vi "test-discretizations.vi"() -> ()   [LabVIEW 2019]
uses:
  <vilib>/Analysis/Matrix/Datatypes/RealMatrix.ctl
  <vilib>/Rock Robotics/WPI/ThirdParty/JAS_Junk/TrajLib/MatBuilder_Create.vi
  <vilib>/Rock Robotics/WPI/ThirdParty/JAS_Junk/TrajLib/MatrixHelper_CoerceSize.vi
  <vilib>/Rock Robotics/WPI/ThirdParty/JAS_Junk/TrajLib/Trajectory_Library.lvlib
  <vilib>/Analysis/Matrix/NI_Matrix.lvlib
panel:
  out "CoVar 2":T1
  out "Cost 1":T1
  # "assertEquals(1.0, mat.get(0, 0), 1e-3);\n    assertEquals(0.0, mat.get(0, 1), 1e-3);\n    assertEquals(0.0, mat.get(0, 2), 1e-3);\n    assertEquals(0.0, mat.get(1, 0), 1e-3);\n    assertEquals(1.0 / 4.0, mat.get(1, 1), 1e-3);\n    assertEquals(0.0, mat.get(1, 2), 1e-3);\n    assertEquals(0.0, mat.get(0, 2), 1e-3);\n    assertEquals(0.0, mat.get(1, 2), 1e-3);\n    assertEquals(1.0 / 9.0, mat.get(2, 2), 1e-3);"
  # "assertEquals(1.0, mat.get(0, 0), 1e-3);\n    assertEquals(0.0, mat.get(0, 1), 1e-3);\n    assertEquals(0.0, mat.get(0, 2), 1e-3)\n;\n    assertEquals(0.0, mat.get(1, 0), 1e-3);\n    assertEquals(4.0, mat.get(1, 1), 1e-3);\n    assertEquals(0.0, mat.get(1, 2), 1e-3);\n\n    assertEquals(0.0, mat.get(0, 2), 1e-3);\n    assertEquals(0.0, mat.get(1, 2), 1e-3);\n    assertEquals(9.0, mat.get(2, 2), 1e-3);"
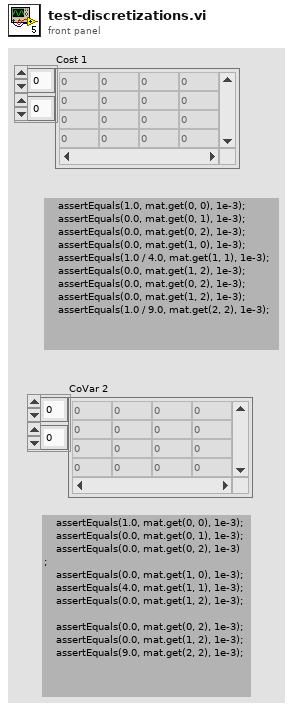
[diagram p1: front panel]
types:
  T1 = typedef "NI_Matrix.lvlib/RealMatrix.ctl" = dbl[][]
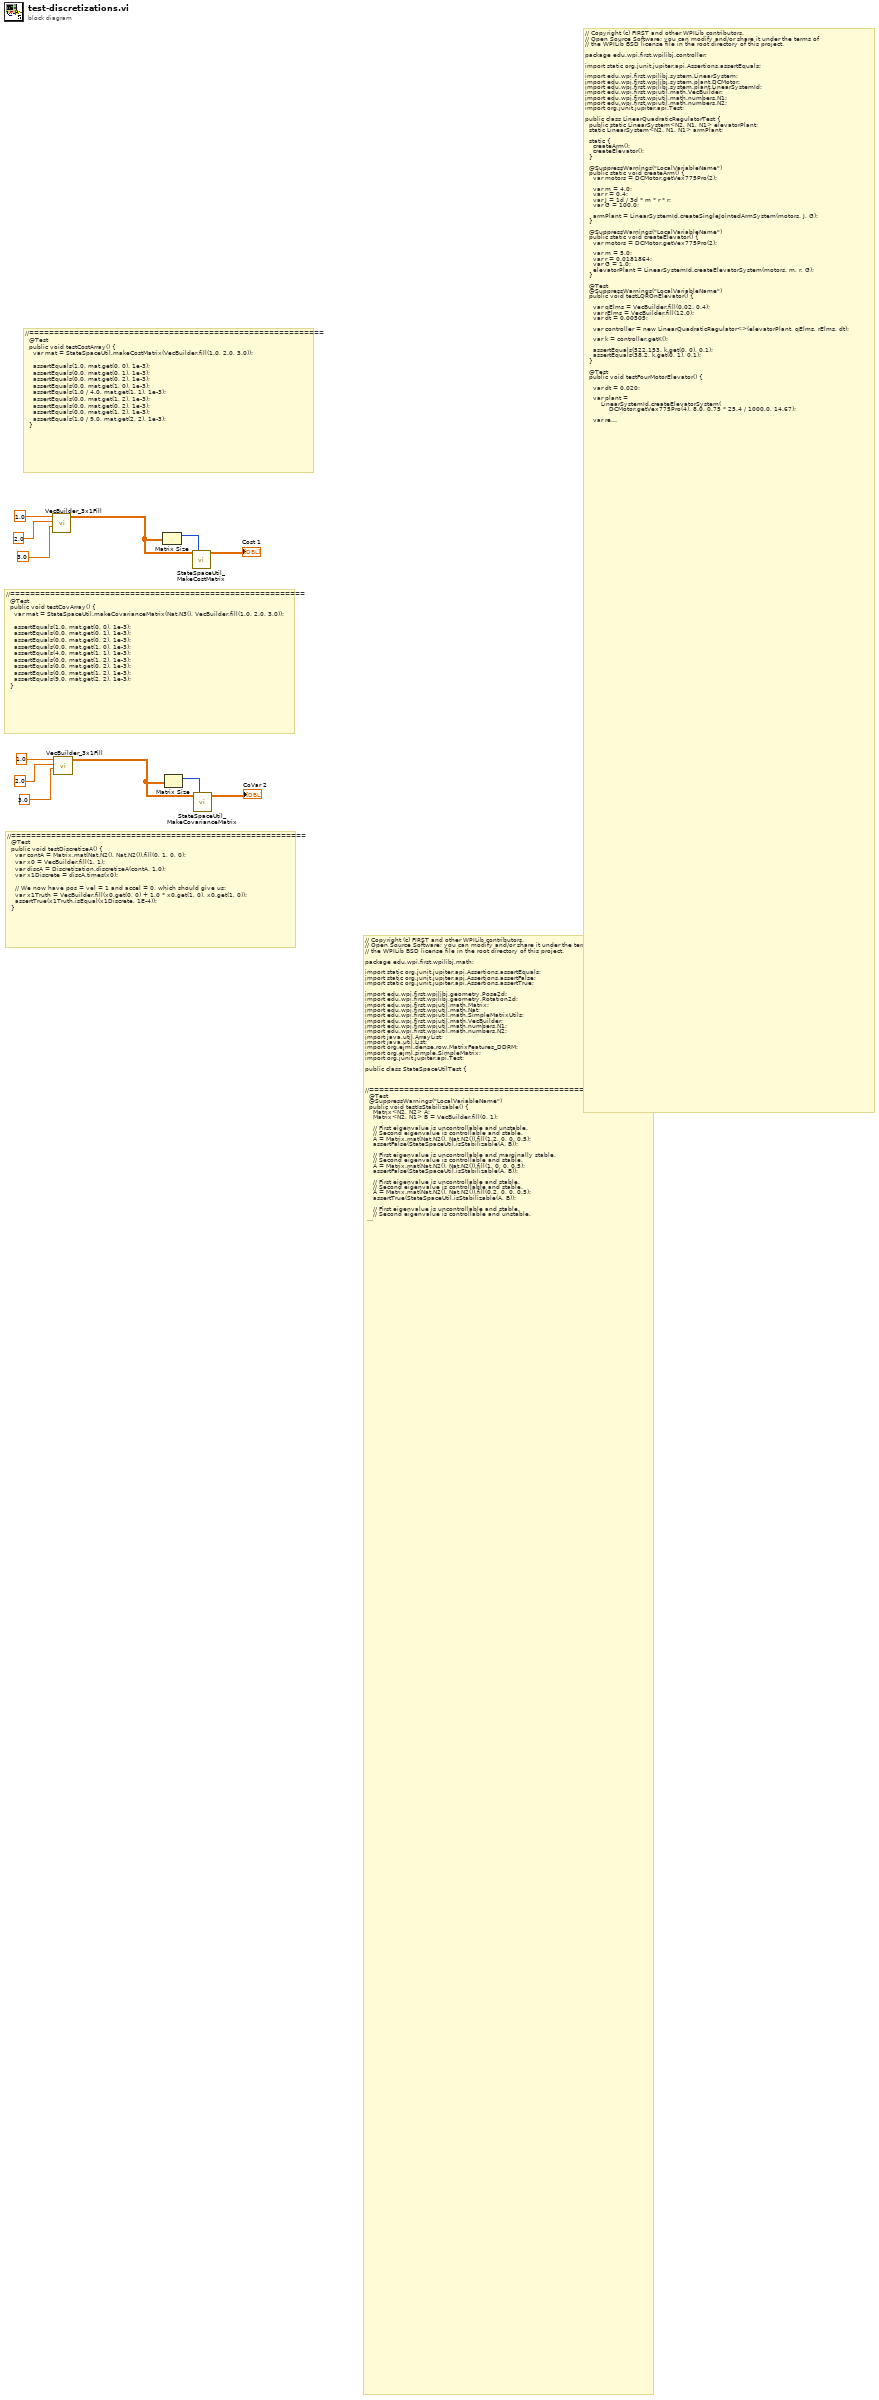
[diagram p0: block diagram]
diagram:
  # "//===========================================================\n  @Test\n  public void testDiscretizeA() {\n    var contA = Matrix.mat(Nat.N2(), Nat.N2()).fill(0, 1, 0, 0);\n    var x0 = VecBuilder.fill(1, 1);\n    var discA = Discretization.discretizeA(contA, 1.0);\n    var x1Discrete = discA.times(x0);\n\n    // We now have pos = vel = 1 and accel = 0, which should give us:\n    var x1Truth = VecBuilder.fill(x0.get(0, 0) + 1.0 * x0.get(1, 0), x0.get(1, 0));\n    assertTrue(x1Truth.isEqual(x1Discrete, 1E-4));\n  }"
  # "//===========================================================\n  @Test\n  public void testCovArray() {\n    var mat = StateSpaceUtil.makeCovarianceMatrix(Nat.N3(), VecBuilder.fill(1.0, 2.0, 3.0));\n\n    assertEquals(1.0, mat.get(0, 0), 1e-3);\n    assertEquals(0.0, mat.get(0, 1), 1e-3);\n    assertEquals(0.0, mat.get(0, 2), 1e-3);\n    assertEquals(0.0, mat.get(1, 0), 1e-3);\n    assertEquals(4.0, mat.get(1, 1), 1e-3);\n    assertEquals(0.0, mat.get(1, 2), 1e-3);\n    assertEquals(0.0, mat.get(0, 2), 1e-3);\n    assertEquals(0.0, mat.get(1, 2), 1e-3);\n    assertEquals(9.0, mat.get(2, 2), 1e-3);\n  }"
  # "//===========================================================\n  @Test\n  public void testCostArray() {\n    var mat = StateSpaceUtil.makeCostMatrix(VecBuilder.fill(1.0, 2.0, 3.0));\n\n    assertEquals(1.0, mat.get(0, 0), 1e-3);\n    assertEquals(0.0, mat.get(0, 1), 1e-3);\n    assertEquals(0.0, mat.get(0, 2), 1e-3);\n    assertEquals(0.0, mat.get(1, 0), 1e-3);\n    assertEquals(1.0 / 4.0, mat.get(1, 1), 1e-3);\n    assertEquals(0.0, mat.get(1, 2), 1e-3);\n    assertEquals(0.0, mat.get(0, 2), 1e-3);\n    assertEquals(0.0, mat.get(1, 2), 1e-3);\n    assertEquals(1.0 / 9.0, mat.get(2, 2), 1e-3);\n  }"
  # "// Copyright (c) FIRST and other WPILib contributors.\n// Open Source Software; you can modify and/or share it under the terms of\n// the WPILib BSD license file in the root directory of this project.\n\npackage edu.wpi.first.wpilibj.math;\n\nimport static org.junit.jupiter.api.Assertions.assertEquals;\nimport static org.junit.jupiter.api.Assertions.assertFalse;\nimport static org.junit.jupiter.api.Assertions.assertTrue;\n\nimport edu.wpi.first.wpilibj.geometry.Pose2d;\nimport edu.wpi.first.wpilibj.geometry.Rotation2d;\nimport edu.wpi.first.wpiutil.math.Matrix;\nimport edu.wpi.first.wpiutil.math.Nat;\nimport edu.wpi.first.wpiutil.math.SimpleMatrixUtils;\nimport edu.wpi.first.wpiutil.math.VecBuilder;\nimport edu.wpi.first.wpiutil.math.numbers.N1;\nimport edu.wpi.first.wpiutil.math.numbers.N2;\nimport java.util.ArrayList;\nimport java.util.List;\nimport org.ejml.dense.row.MatrixFeatures_DDRM;\nimport org.ejml.simple.SimpleMatrix;\nimport org.junit.jupiter.api.Test;\n\npublic class StateSpaceUtilTest {\n\n\n\n//===========================================================\n  @Test\n  @SuppressWarnings(\"LocalVariableName\")\n  public void testIsStabilizable() {\n    Matrix<N2, N2> A;\n    Matrix<N2, N1> B = VecBuilder.fill(0, 1);\n\n    // First eigenvalue is uncontrollable and unstable.\n    // Second eigenvalue is controllable and stable.\n    A = Matrix.mat(Nat.N2(), Nat.N2()).fill(1.2, 0, 0, 0.5);\n    assertFalse(StateSpaceUtil.isStabilizable(A, B));\n\n    // First eigenvalue is uncontrollable and marginally stable.\n    // Second eigenvalue is controllable and stable.\n    A = Matrix.mat(Nat.N2(), Nat.N2()).fill(1, 0, 0, 0.5);\n    assertFalse(StateSpaceUtil.isStabilizable(A, B));\n\n    // First eigenvalue is uncontrollable and stable.\n    // Second eigenvalue is controllable and stable.\n    A = Matrix.mat(Nat.N2(), Nat.N2()).fill(0.2, 0, 0, 0.5);\n    assertTrue(StateSpaceUtil.isStabilizable(A, B));\n\n    // First eigenvalue is uncontrollable and stable.\n    // Second eigenvalue is controllable and unstable.\n    A = Matrix.mat(Nat.N2(), Nat.N2()).fill(0.2, 0, 0, 1.2);\n    assertTrue(StateSpaceUtil.isStabilizable(A, B));\n  }\n\n//===========================================================\n  @Test\n  public void testMakeWhiteNoiseVector() {\n    var firstData = new ArrayList<Double>();\n    var secondData = new ArrayList<Double>();\n    for (int i = 0; i < 1000; i++) {\n      var noiseVec = StateSpaceUtil.makeWhiteNoiseVector(VecBuilder.fill(1.0, 2.0));\n      firstData.add(noiseVec.get(0, 0));\n      secondData.add(noiseVec.get(1, 0));\n    }\n    assertEquals(1.0, calculateStandardDeviation(firstData), 0.2);\n    assertEquals(2.0, calculateStandardDeviation(secondData), 0.2);\n  }\n\n  private double calculateStandardDeviation(List<Double> numArray) {\n    double sum = 0.0;\n    double standardDeviation = 0.0;\n    int length = numArray.size();\n\n    for (double num : numArray) {\n      sum += num;\n    }\n\n    double mean = sum / length;\n\n    for (double num : numArray) {\n      standardDeviation += Math.pow(num - mean, 2);\n    }\n\n    return Math.sqrt(standardDeviation / length);\n  }\n\n\n//===========================================================\n  @SuppressWarnings(\"LocalVariableName\")\n  @Test\n  public void testDiscretizeAB() {\n    var contA = Matrix.mat(Nat.N2(), Nat.N2()).fill(0, 1, 0, 0);\n    var contB = VecBuilder.fill(0, 1);\n    var x0 = VecBuilder.fill(1, 1);\n    var u = VecBuilder.fill(1);\n\n    var abPair = Discretization.discretizeAB(contA, contB, 1.0);\n\n    var x1Discrete = abPair.getFirst().times(x0).plus(abPair.getSecond().times(u));\n\n    // We now have pos = vel = accel = 1, which should give us:\n    var x1Truth =\n        VecBuilder.fill(\n            x0.get(0, 0) + x0.get(1, 0) + 0.5 * u.get(0, 0), x0.get(0, 0) + u.get(0, 0));\n\n    assertTrue(x1Truth.isEqual(x1Discrete, 1E-4));\n  }\n\n//===========================================================\n  @Test\n  public void testMatrixExp() {\n    Matrix<N2, N2> wrappedMatrix = Matrix.eye(Nat.N2());\n    var wrappedResult = wrappedMatrix.exp();\n\n    assertTrue(\n        wrappedResult.isEqual(Matrix.mat(Nat.N2(), Nat.N2()).fill(Math.E, 0, 0, Math.E), 1E-9));\n\n    var matrix = Matrix.mat(Nat.N2(), Nat.N2()).fill(1, 2, 3, 4);\n    wrappedResult = matrix.times(0.01).exp();\n\n    assertTrue(\n        wrappedResult.isEqual(\n            Matrix.mat(Nat.N2(), Nat.N2()).fill(1.01035625, 0.02050912, 0.03076368, 1.04111993),\n            1E-8));\n  }\n\n//===========================================================\n  @Test\n  public void testSimpleMatrixExp() {\n    SimpleMatrix matrix = SimpleMatrixUtils.eye(2);\n    var result = SimpleMatrixUtils.exp(matrix);\n\n    assertTrue(\n        MatrixFeatures_DDRM.isIdentical(\n            result.getDDRM(),\n            new SimpleMatrix(2, 2, true, new double[] {Math.E, 0, 0, Math.E}).getDDRM(),\n            1E-9));\n\n    matrix = new SimpleMatrix(2, 2, true, new double[] {1, 2, 3, 4});\n    result = SimpleMatrixUtils.exp(matrix.scale(0.01));\n\n    assertTrue(\n        MatrixFeatures_DDRM.isIdentical(\n            result.getDDRM(),\n            new SimpleMatrix(\n                    2, 2, true, new double[] {1.01035625, 0.02050912, 0.03076368, 1.04111993})\n                .getDDRM(),\n            1E-8));\n  }\n\n//===========================================================\n  @Test\n  public void testPoseToVector() {\n    Pose2d pose = new Pose2d(1, 2, new Rotation2d(3));\n    var vector = StateSpaceUtil.poseToVector(pose);\n    assertEquals(pose.getTranslation().getX(), vector.get(0, 0), 1e-6);\n    assertEquals(pose.getTranslation().getY(), vector.get(1, 0), 1e-6);\n    assertEquals(pose.getRotation().getRadians(), vector.get(2, 0), 1e-6);\n  }\n}"
  # "// Copyright (c) FIRST and other WPILib contributors.\n// Open Source Software; you can modify and/or share it under the terms of\n// the WPILib BSD license file in the root directory of this project.\n\npackage edu.wpi.first.wpilibj.controller;\n\nimport static org.junit.jupiter.api.Assertions.assertEquals;\n\nimport edu.wpi.first.wpilibj.system.LinearSystem;\nimport edu.wpi.first.wpilibj.system.plant.DCMotor;\nimport edu.wpi.first.wpilibj.system.plant.LinearSystemId;\nimport edu.wpi.first.wpiutil.math.VecBuilder;\nimport edu.wpi.first.wpiutil.math.numbers.N1;\nimport edu.wpi.first.wpiutil.math.numbers.N2;\nimport org.junit.jupiter.api.Test;\n\npublic class LinearQuadraticRegulatorTest {\n  public static LinearSystem<N2, N1, N1> elevatorPlant;\n  static LinearSystem<N2, N1, N1> armPlant;\n\n  static {\n    createArm();\n    createElevator();\n  }\n\n  @SuppressWarnings(\"LocalVariableName\")\n  public static void createArm() {\n    var motors = DCMotor.getVex775Pro(2);\n\n    var m = 4.0;\n    var r = 0.4;\n    var J = 1d / 3d * m * r * r;\n    var G = 100.0;\n\n    armPlant = LinearSystemId.createSingleJointedArmSystem(motors, J, G);\n  }\n\n  @SuppressWarnings(\"LocalVariableName\")\n  public static void createElevator() {\n    var motors = DCMotor.getVex775Pro(2);\n\n    var m = 5.0;\n    var r = 0.0181864;\n    var G = 1.0;\n    elevatorPlant = LinearSystemId.createElevatorSystem(motors, m, r, G);\n  }\n\n  @Test\n  @SuppressWarnings(\"LocalVariableName\")\n  public void testLQROnElevator() {\n\n    var qElms = VecBuilder.fill(0.02, 0.4);\n    var rElms = VecBuilder.fill(12.0);\n    var dt = 0.00505;\n\n    var controller = new LinearQuadraticRegulator<>(elevatorPlant, qElms, rElms, dt);\n\n    var k = controller.getK();\n\n    assertEquals(522.153, k.get(0, 0), 0.1);\n    assertEquals(38.2, k.get(0, 1), 0.1);\n  }\n\n  @Test\n  public void testFourMotorElevator() {\n\n    var dt = 0.020;\n\n    var plant =\n        LinearSystemId.createElevatorSystem(\n            DCMotor.getVex775Pro(4), 8.0, 0.75 * 25.4 / 1000.0, 14.67);\n\n    var regulator =\n        new LinearQuadraticRegulator<>(plant, VecBuilder.fill(0.1, 0.2), VecBuilder.fill(12.0), dt);\n\n    assertEquals(10.381, regulator.getK().get(0, 0), 1e-2);\n    assertEquals(0.6929, regulator.getK().get(0, 1), 1e-2);\n  }\n\n  @Test\n  @SuppressWarnings(\"LocalVariableName\")\n  public void testLQROnArm() {\n\n    var motors = DCMotor.getVex775Pro(2);\n\n    var m = 4.0;\n    var r = 0.4;\n    var G = 100.0;\n\n    var plant = LinearSystemId.createSingleJointedArmSystem(motors, 1d / 3d * m * r * r, G);\n\n    var qElms = VecBuilder.fill(0.01745, 0.08726);\n    var rElms = VecBuilder.fill(12.0);\n    var dt = 0.00505;\n\n    var controller = new LinearQuadraticRegulator<>(plant, qElms, rElms, dt);\n\n    var k = controller.getK();\n\n    assertEquals(19.16, k.get(0, 0), 0.1);\n    assertEquals(3.32, k.get(0, 1), 0.1);\n  }\n\n  @Test\n  public void testLatencyCompensate() {\n    var dt = 0.02;\n\n    var plant =\n        LinearSystemId.createElevatorSystem(\n            DCMotor.getVex775Pro(4), 8.0, 0.75 * 25.4 / 1000.0, 14.67);\n\n    var regulator =\n        new LinearQuadraticRegulator<>(plant, VecBuilder.fill(0.1, 0.2), VecBuilder.fill(12.0), dt);\n\n    regulator.latencyCompensate(plant, dt, 0.01);\n\n    assertEquals(8.97115941, regulator.getK().get(0, 0), 1e-3);\n    assertEquals(0.07904881, regulator.getK().get(0, 1), 1e-3);\n  }\n}"
  n1 = call <vilib>:"VecBuilder_3x1Fill.vi"("R2"=3.0, "R1"=2.0, "R0"=1.0) -> ("output matrix"=w10:T1)  [unwired: 8 in]
  n2 = call <vilib>:"VecBuilder_3x1Fill.vi"("R2"=3.0, "R1"=2.0, "R0"=1.0) -> ("output matrix"=w4:T1)  [unwired: 8 in]
  n3 = Matrix Size(0:w10) -> (1:w9:i32)  [unwired: 1 out]
  n4 = Matrix Size(0:w4) -> (1:w3:i32)  [unwired: 1 out]
  n5 = call <vilib>:"StateSpaceUtil_MakeCostMatrix.vi"("States"=w9, "Costs"=w10) -> ("Costs Matrix"=→"Cost 1":T1)  [unwired: 9 in]
  n6 = call <vilib>:"StateSpaceUtil_MakeCovarianceMatrix.vi"("States"=w3, "StdDevs"=w4) -> ("Covariance Matrix"=→"CoVar 2":T1)  [unwired: 9 in]
